vi "Untitled 3.vi"() -> ()   [LabVIEW 2017]
uses:
  <vilib>/myRIO/Instrument Drivers/Onboard IO/AI/typedefs/AI Reference.ctl
  <vilib>/myRIO/Common/Instrument Driver Framework/Utilities/typedefs/myRIO Generic Hardware Reference.ctl
  <vilib>/myRIO/Common/Instrument Driver Framework/Utilities/typedefs/Hardware Version Enum.ctl
  <vilib>/myRIO/Common/Instrument Driver Framework/Utilities/typedefs/myRIO v1.0 Reference.ctl
  <vilib>/myRIO/Common/Instrument Driver Framework/Utilities/typedefs/Generic FPGA Reference.ctl
  <vilib>/myRIO/Common/Instrument Driver Framework/myRIO v1.0/AI/typedefs/AI Channels List.ctl
  <vilib>/myRIO/Common/Instrument Driver Framework/myRIO v1.0/AI/typedefs/AI Channels Enum.ctl
  <vilib>/myRIO/Common/Instrument Driver Framework/Utilities/typedefs/Analog Scaling Constants List.ctl
  <vilib>/myRIO/Common/Instrument Driver Framework/Utilities/typedefs/Analog Scaling Constants.ctl
  <vilib>/userdefined/High Color/nirio_resource_hc.ctl
  <vilib>/myRIO/Common/Instrument Driver Framework/Utilities/vis/Is FPGA Ref Available.vi
  <vilib>/myRIO/Common/Instrument Driver Framework/myRIO v1.0/AI/vis/myRIO v1.1 Open AI.vi
  <vilib>/myRIO/Instrument Drivers/Onboard IO/AI/vis/Read.vi
  <vilib>/myRIO/Common/Instrument Driver Framework/Utilities/vis/Validate Channels.vi
  <vilib>/myRIO/Common/Instrument Driver Framework/myRIO v1.0/AI/vis/myRIO v1.0 Reserve AI.vi
  <vilib>/myRIO/Common/Instrument Driver Framework/myRIO v1.0/AI/vis/myRIO v1.0 Build MUX Configuration AI.vi
  <vilib>/myRIO/Common/Instrument Driver Framework/myRIO v1.0/Resource Manager/vis/myRIO v1.0 Reserve Channel List.vi
  <vilib>/myRIO/Common/Instrument Driver Framework/myRIO v1.0/Resource Manager/vis/myRIO v1.0 Reserve Channel.vi
  <vilib>/myRIO/Common/Instrument Driver Framework/myRIO v1.0/Resource Manager/vis/myRIO v1.0 Unreserve Channel.vi
  <vilib>/myRIO/Common/Instrument Driver Framework/myRIO v1.0/Resource Manager/vis/myRIO v1.0 Build Mutex Name.vi
  <vilib>/Utility/VariantDataType/GetNumericInfo.vi
  <vilib>/Utility/error.llb/Error Cluster From Error Code.vi
  <vilib>/myRIO/Common/Instrument Driver Framework/myRIO v1.0/myRIO v1.1 Open.vi
  <vilib>/myRIO/Common/Instrument Driver Framework/myRIO v1.0/AI/vis/myRIO v1.0 Get Scaling Constants AI.vi
  <vilib>/myRIO/Common/Instrument Driver Framework/Utilities/vis/IO Manager.vi
  <vilib>/myRIO/Common/Instrument Driver Framework/Utilities/vis/Configuration Manager.vi
  <vilib>/myRIO/Common/Instrument Driver Framework/myRIO v1.0/myRIO v1.0 Close.vi
  <vilib>/myRIO/Common/Instrument Driver Framework/myRIO v1.0/AI/vis/myRIO v1.0 Read AI.vi
  <vilib>/myRIO/Express VI/Onboard IO/AI/AI Express VI.xnode
  <vilib>/myRIO/Instrument Drivers/Onboard IO/AI/vis/myRIO AI Open.xnode
  <vilib>/myRIO/Instrument Drivers/Onboard IO/AI/AI.lvlib
panel:
  in  "stop":bool
  out "Waveform Chart":dbl(graph)
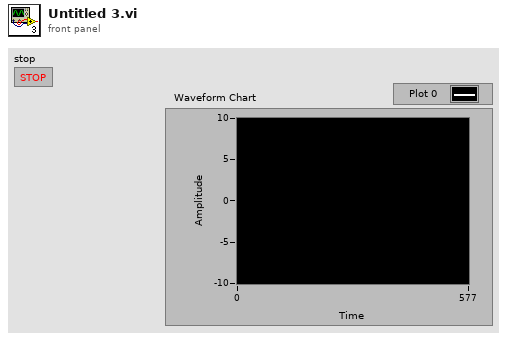
[diagram p1: front panel]
types:
  T1 = typedef "AI.lvlib/AI Reference.ctl" = cluster{"myRIO Reference":T2, "AI Channels List":T6, "AI Scaling Constants List":T8}
  T2 = typedef "myRIO Generic Hardware Reference.ctl" = cluster{"myRIO Model":T3, "myRIO Hardware Reference":T4}
  T3 = typedef "Hardware Version Enum.ctl" = enum16{"Unknown", "myRIO-1900", "myRIO-1950", "roboRIO", "NI ELVIS RIO CM"}
  T4 = typedef "myRIO v1.0 Reference.ctl" = cluster{"Generic FPGA Reference":T5, "Allow multiple opens":bool}
  T5 = typedef "Generic FPGA Reference.ctl" = refnum<k20>
  T6 = typedef "AI Channels List.ctl" = T7[]
  T7 = typedef "AI Channels Enum.ctl" = enum16{"Not Connected", "AudioIn/Left", "AudioIn/Right", "C/AI0", "C/AI1", "A/AI0", "A/AI1", "A/AI2", "A/AI3", "B/AI0", "B/AI1", "B/AI2", "B/AI3", "AI/AI0", "AI/AI1", "AI/AI2", "AI/AI3"}
  T8 = typedef "Analog Scaling Constants List.ctl" = T9[]
  T9 = typedef "Analog Scaling Constants.ctl" = cluster{"LSB Weight (Volts)":dbl, "Offset (Volts)":dbl, "Signed?":bool}
  T10 = typedef "nirio_resource_hc.ctl" = tag
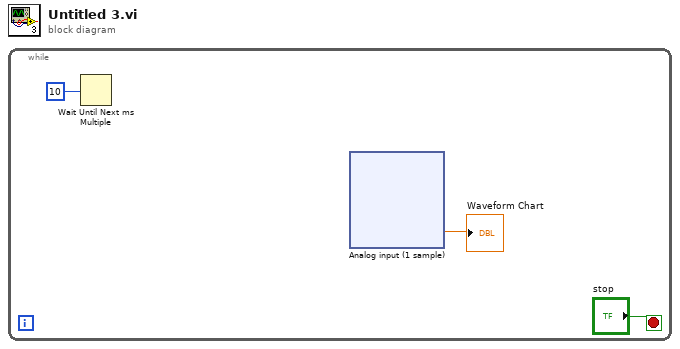
[diagram p0: block diagram]
diagram:
  n1 = while {
    stop <- "stop" stop-if-true
    n2 = Wait Until Next ms Multiple(millisecond multiple=u32 10 ("millisecond timer value")) -> ()  [unwired: 1 out]
    n3 = xnode "Analog input (1 sample)"() -> ("C/AI0 (AI0)"=→"Waveform Chart":dbl)  [unwired: 1 in, 1 out]
  }
